vi "check end.vi"(11 "input plate":u8[][](array[numeric])) -> ()   [LabVIEW 2024]
panel:
  out "Highest":u8
  out "End?":bool
  in  "buf block style":u8[](array[numeric])
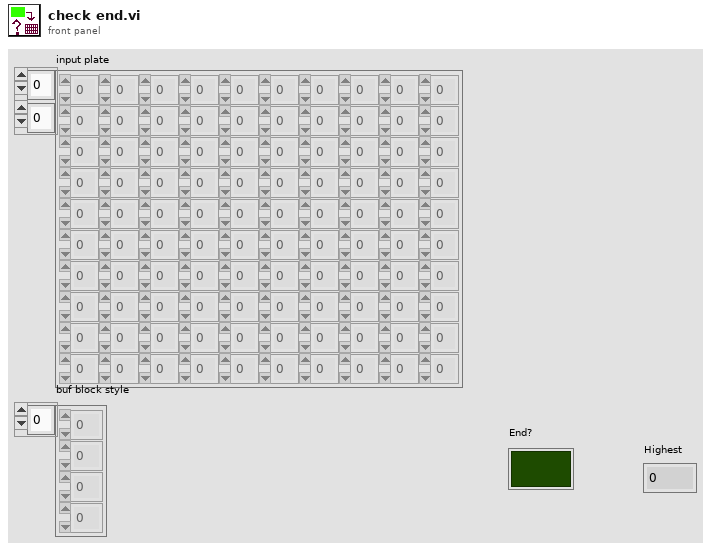
[diagram p1: front panel]
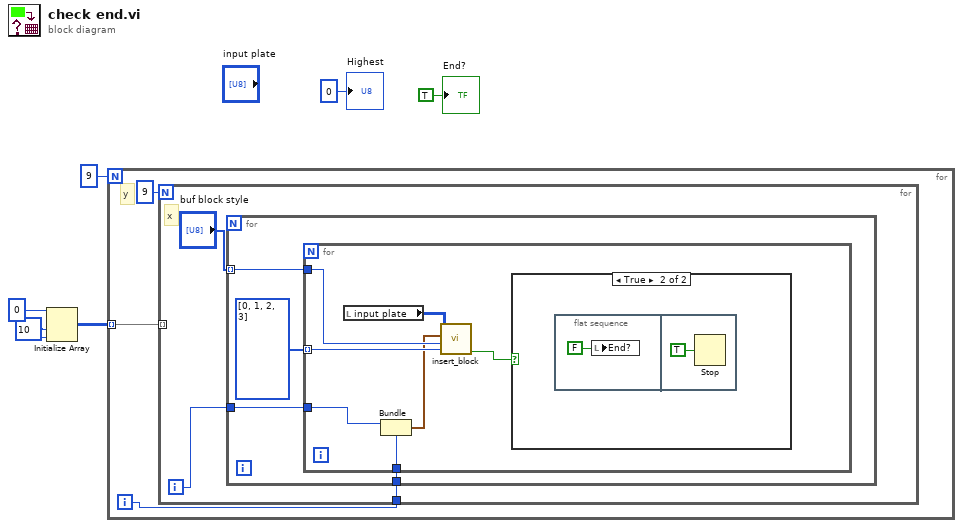
[diagram p0: block diagram]
diagram:
  w6 = 10 ("dimension size")
  n1 = Initialize Array(u32 0 ("element"), w6, w6) -> (w3:u32[][])
  n2 = for {
    N: 9 -> [_]
    tunnel: w3 -> [w8] mode=indexing
    i -> [w7]
    # "y"
    n3 = for {
      N: 9 -> [_]
      tunnel: w8 -> [_] mode=indexing
      tunnel: w7 -> [w11]
      i -> [w12]
      # "x"
      n4 = for {
        tunnel: w12 -> [w16]
        tunnel: w11 -> [w15]
        tunnel: "buf block style" -> [w13] mode=indexing
        n5 = for {
          tunnel: w16 -> [w22]
          tunnel: w15 -> [w21]
          tunnel: u16[] [0, 1, 2, 3] -> [w20] mode=indexing
          tunnel: w13 -> [w19]
          n6 = local read "input plate"() -> (w23:u8[][])
          n7 = Bundle(w22, w21) -> (w18:cluster{i32, i32})  [unwired: 1 in]
          n8 = call "insert_block.vi"("direction"=w20, "block_type"=w19, "position"=w18, "plate arr"=w23) -> ("valid?"=w17:bool)  [unwired: 6 in, 1 out]
          n9 = case shown="True" w17 {
            frame False {
            }
            frame True {
              n10 = flat-sequence {
                frame #0 {
                  n11 = local write "End?"(FALSE ("End?")) -> ()
                }
                frame #1 {
                  n12 = Stop(stop? (T)=TRUE) -> ()
                }
              }
            }
          }
        }
      }
    }
  }
  "End?" <- TRUE ("End?")
  "Highest" <- u8 0 ("Highest")
